vi "Track Debug Event.vi"(8 "error in (no error)":errorcluster, 10 "Debug Data.lvclass":refnum<class "Debug Data.lvclass">, 11 "Debug Latest Message In":refnum<class "Debug Latest Broadcast.lvclass">) -> (0 "error out":errorcluster, 3 "Debug Latest Message Out":refnum<class "Debug Latest Broadcast.lvclass">)   [LabVIEW 2020, in "Debug Latest Broadcast.lvclass"]
uses:
  Debug Latest Broadcast.lvclass
  Debug Data/Debug Data.lvclass
  Debug Data/Debug Data.lvclass/Debug Data.ctl
  Debug Latest Broadcast.lvclass/Debug Latest Broadcast.ctl
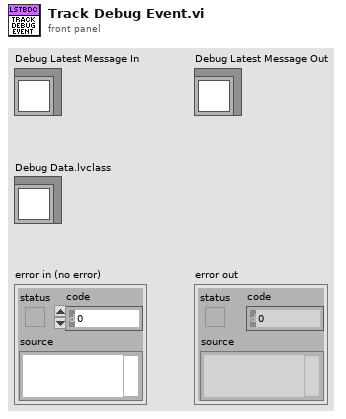
[diagram p1: front panel]
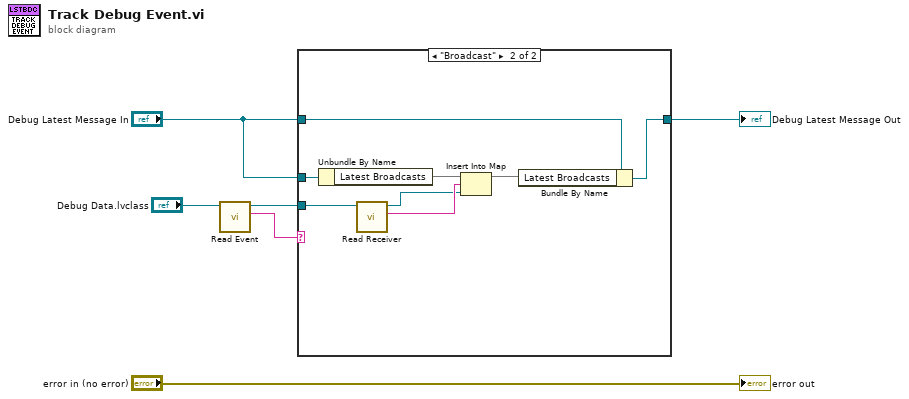
[diagram p0: block diagram]
diagram:
  n1 = call "Read Event.vi"("Debug Data in"="Debug Data.lvclass") -> ("Event"=w4:string, "Debug Data out"=w3:refnum<class "Debug Data.lvclass">)  [unwired: 9 in]
  n2 = case shown="\"Broadcast\"" w4 {
    tunnel: w3 -> [_ w13]
    tunnel: "Debug Latest Message In" -> [_ w15]
    tunnel: "Debug Latest Message In" -> [w7 w10]
    tunnel: [w7 w8] -> w1
    frame Default {
    }
    frame "Broadcast" {
      n3 = Unbundle By Name(w15) -> ("Latest Broadcasts"=w14:map{string, refnum<class "Debug Data.lvclass">})
      n4 = call "Read Receiver.vi"("Debug Data In"=w13) -> ("Receiver"=w12:string, "Debug Data Out"=w11:refnum<class "Debug Data.lvclass">)  [unwired: 9 in]
      n5 = Insert Into Map(map in=w14, key=w12, value=w11) -> (map out=w9:map{string, refnum<class "Debug Data.lvclass">})  [unwired: 2 out]
      n6 = Bundle By Name(cluster=w10, "Latest Broadcasts"=w9) -> (w8:refnum<class "Debug Latest Broadcast.lvclass">)
    }
  }
  "Debug Latest Message Out" <- w1
  "error out" <- "error in (no error)"
